vi "FGGA Serial Data Server & Recordingv5.0_10Hz_Scroll_Pump.vi"(0 "VISA resource name out":refnum<visa-resource-name>, 11 "error IO":errorcluster) -> ()   [LabVIEW 2014]
uses:
  <vilib>/Platform/TimedLoop/XDataNode/timing_clust.ctl
  <vilib>/Platform/TimedLoop/XDataNode/nitl_modes.ctl
  <vilib>/Platform/TimedLoop/XDataNode/wakeup.ctl
  C:/Program Files (x86)/National Instruments/LabVIEW 2014/examples/Data Communication/Network Streams/Simple Network Streams/support/Network Stream Command.ctl
  <vilib>/Utility/error.llb/whitespace.ctl
  <vilib>/Utility/tcp.llb/UDP Multicast Write-Only Open.vi
  <vilib>/Instr/_visa.llb/VISA Configure Serial Port (Instr).vi
  <vilib>/platform/TimedLoop/XDataNode/XDataNode.xnode
  <vilib>/Platform/TimedLoop/XDataNode/XDNodeRunTimeDep.lvlib
panel:
  out "FLOW ALL OFF":bool
  out "LOW FLOW MASTER SWITCH":bool
  out "HIGH FLOW MASTER SWITCH":bool
  out "UDP_ASCII_File":string
  out "V12":bool
  out "V11":bool
  out "V10":bool
  out "FGGA Pump":bool
  out "Flight Number":string
  out "Stop File Write":bool
  out "Default file name":string
  out "MFC":dbl[](array[numeric])
  out "FGGA restart":bool
  out "V4":bool
  out "V3":bool
  out "V2":bool
  out "V1":bool
  out "error out 2":errorcluster
  out "error out":errorcluster
  in  "MFC_1 SLPM set value":dbl
  out "Value Read":string
  out "status":bool
  in  "VISA resource name":refnum<visa-resource-name>="ASRL3::INSTR"
  in  "timeout (10sec) 2":u32=3000
  out "Labview_Viewer_UDP_Error_Out":errorcluster
  in  "Clear Display\nErrors":bool
  out "Data Processing":bool
  out "TCP Binary Packet":string
  out "UDP Time Stamp Offset":i32=1
  out "Data String":string
  out "UDP_ACSII_Out":string
  out "Serial error out":errorcluster
  out "SEPTIC TCP Error Out":errorcluster
  out "TCP packet\nSend To SEPTIC":bool
  out "FISH TCP Error Out":errorcluster
  out "TCP packet\nSend To FISH":bool
  out "UDP_Pack_num":u32
  out "UDP_Out Status":bool
  out "UDP_Out_Error Out":errorcluster
  out "Data Array":string[](array[string])
  out "RAW DATA":string
  in  "stop":bool
  out "Number of times \nRead time out":u32
  out "Loop count":i32
  # "Date"
  # "Time"
  # "CH4"
  # "CO2"
  # "H2O"
  # "Cell Pressure"
  # "Cell Temperature"
  # "Spectral Flag"
  # "Ring Down Time (Laser A)"
  # "Ring Down Time (Laser B)"
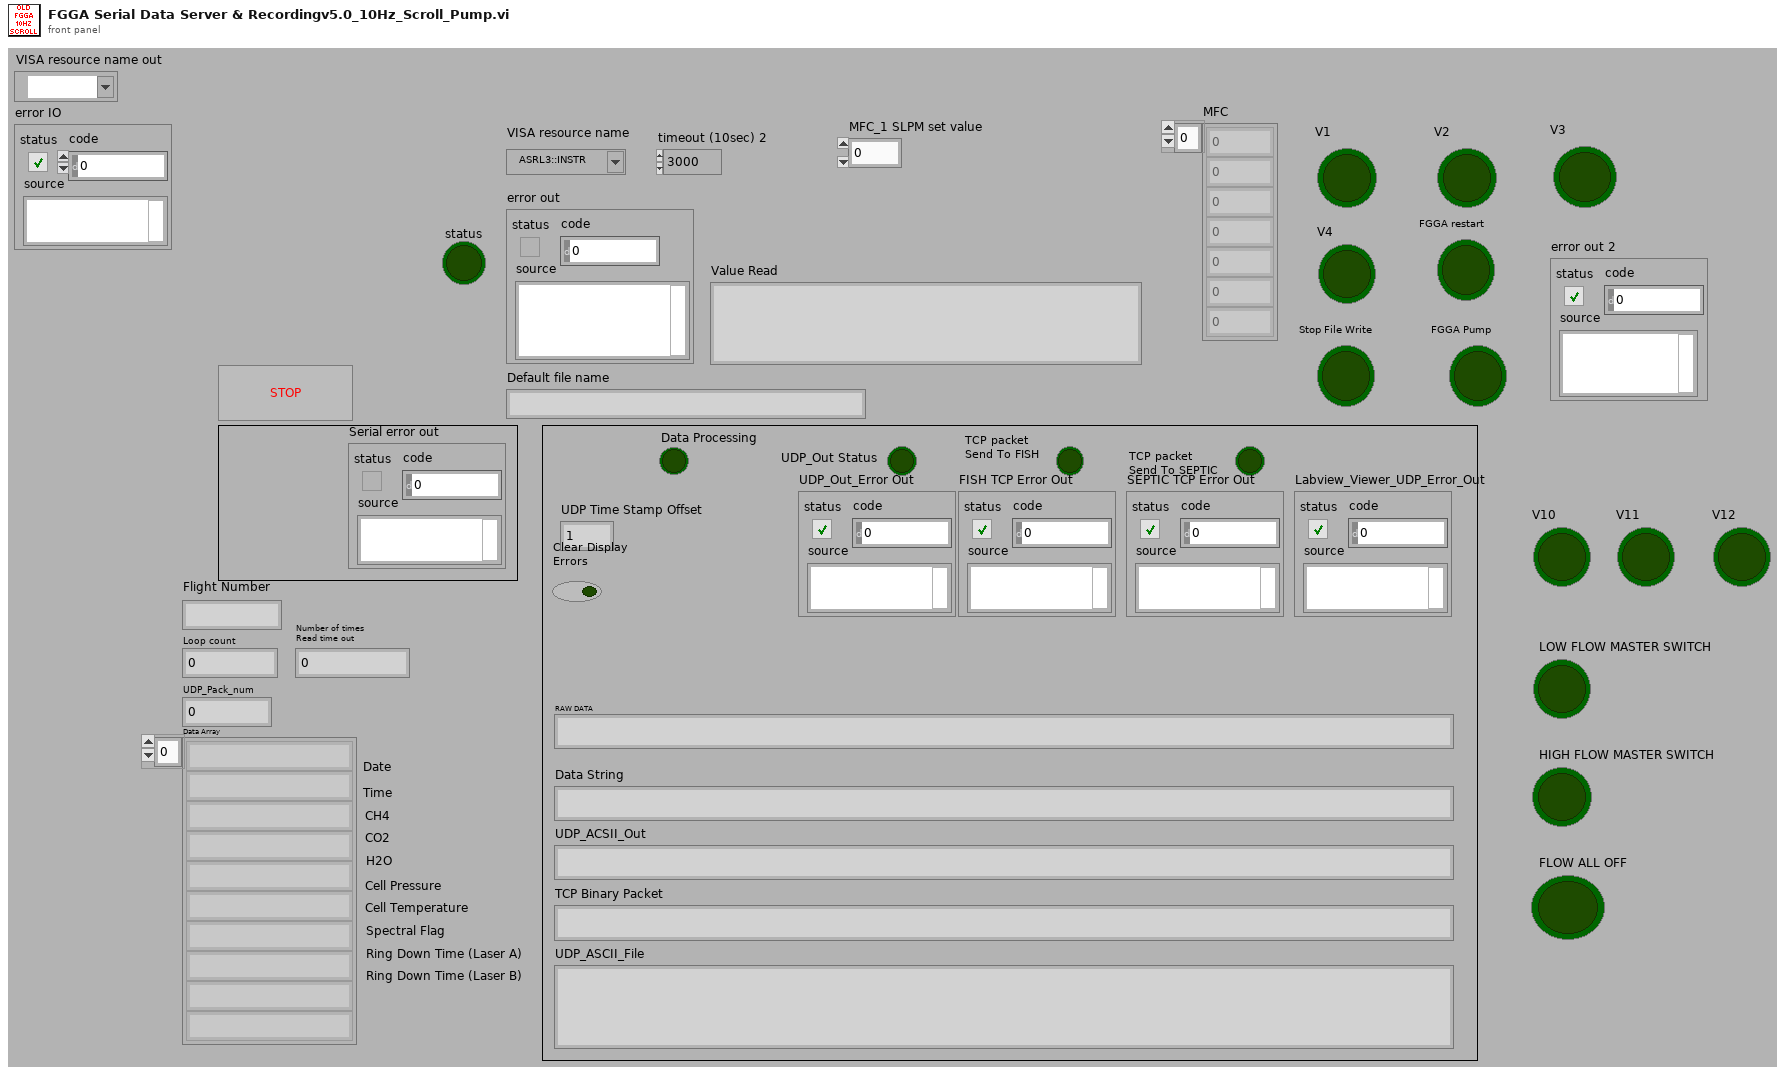
[diagram p1: front panel]
types:
  T1 = typedef "XDNodeRunTimeDep.lvlib/timing_clust.ctl" = cluster{"Expected End [f-1]":u64, "Actual End [f-1]":u64, "Finished Late? [f-1]":bool, "Expected End [i-1]":u64, "Actual End [i-1]":u64, "Finished Late? [i-1]":bool, "Expected Start [i]":u64, "Actual Start [i]":u64, "Expected Start [f]":u64, "Actual Start [f]":u64, "Source Name":string, "Structure Name":string, "Period":i64, "Deadline":i64, "Offset":i64, "Start":i64, "Priority":i32, "Timeout":i32, "Mode":T2, "Wakeup Reason":T3, "Error":errorcluster, "Source Type":string, "Secondary Source Type":string, "Global End Time":u64, "Global Start Time":u64, "Frame Duration":u64, "Iteration Duration":u64, "Assigned CPU":i32, "I/O Scan Engine Mode":u32}
  T2 = typedef "XDNodeRunTimeDep.lvlib/nitl_modes.ctl" = enum32{"No Change", "Process missed periods, maintain original phase", "Discard missed periods, maintain original phase", "Process missed periods, ignore original phase", "Discard missed periods, ignore original phase"}
  T3 = typedef "XDNodeRunTimeDep.lvlib/wakeup.ctl" = enum32{"Normal", "Aborted", "Asynchronous wakeup", "Timing source error", "Timed loop error", "Timeout"}
  T4 = typedef "Network Stream Command.ctl" = cluster{"Message":string, "Message Data":variant}
  T5 = enum16{"open", "replace", "create", "open or create", "replace or create", "replace or create with confirmation"}
  T6 = typedef "whitespace.ctl" = u16
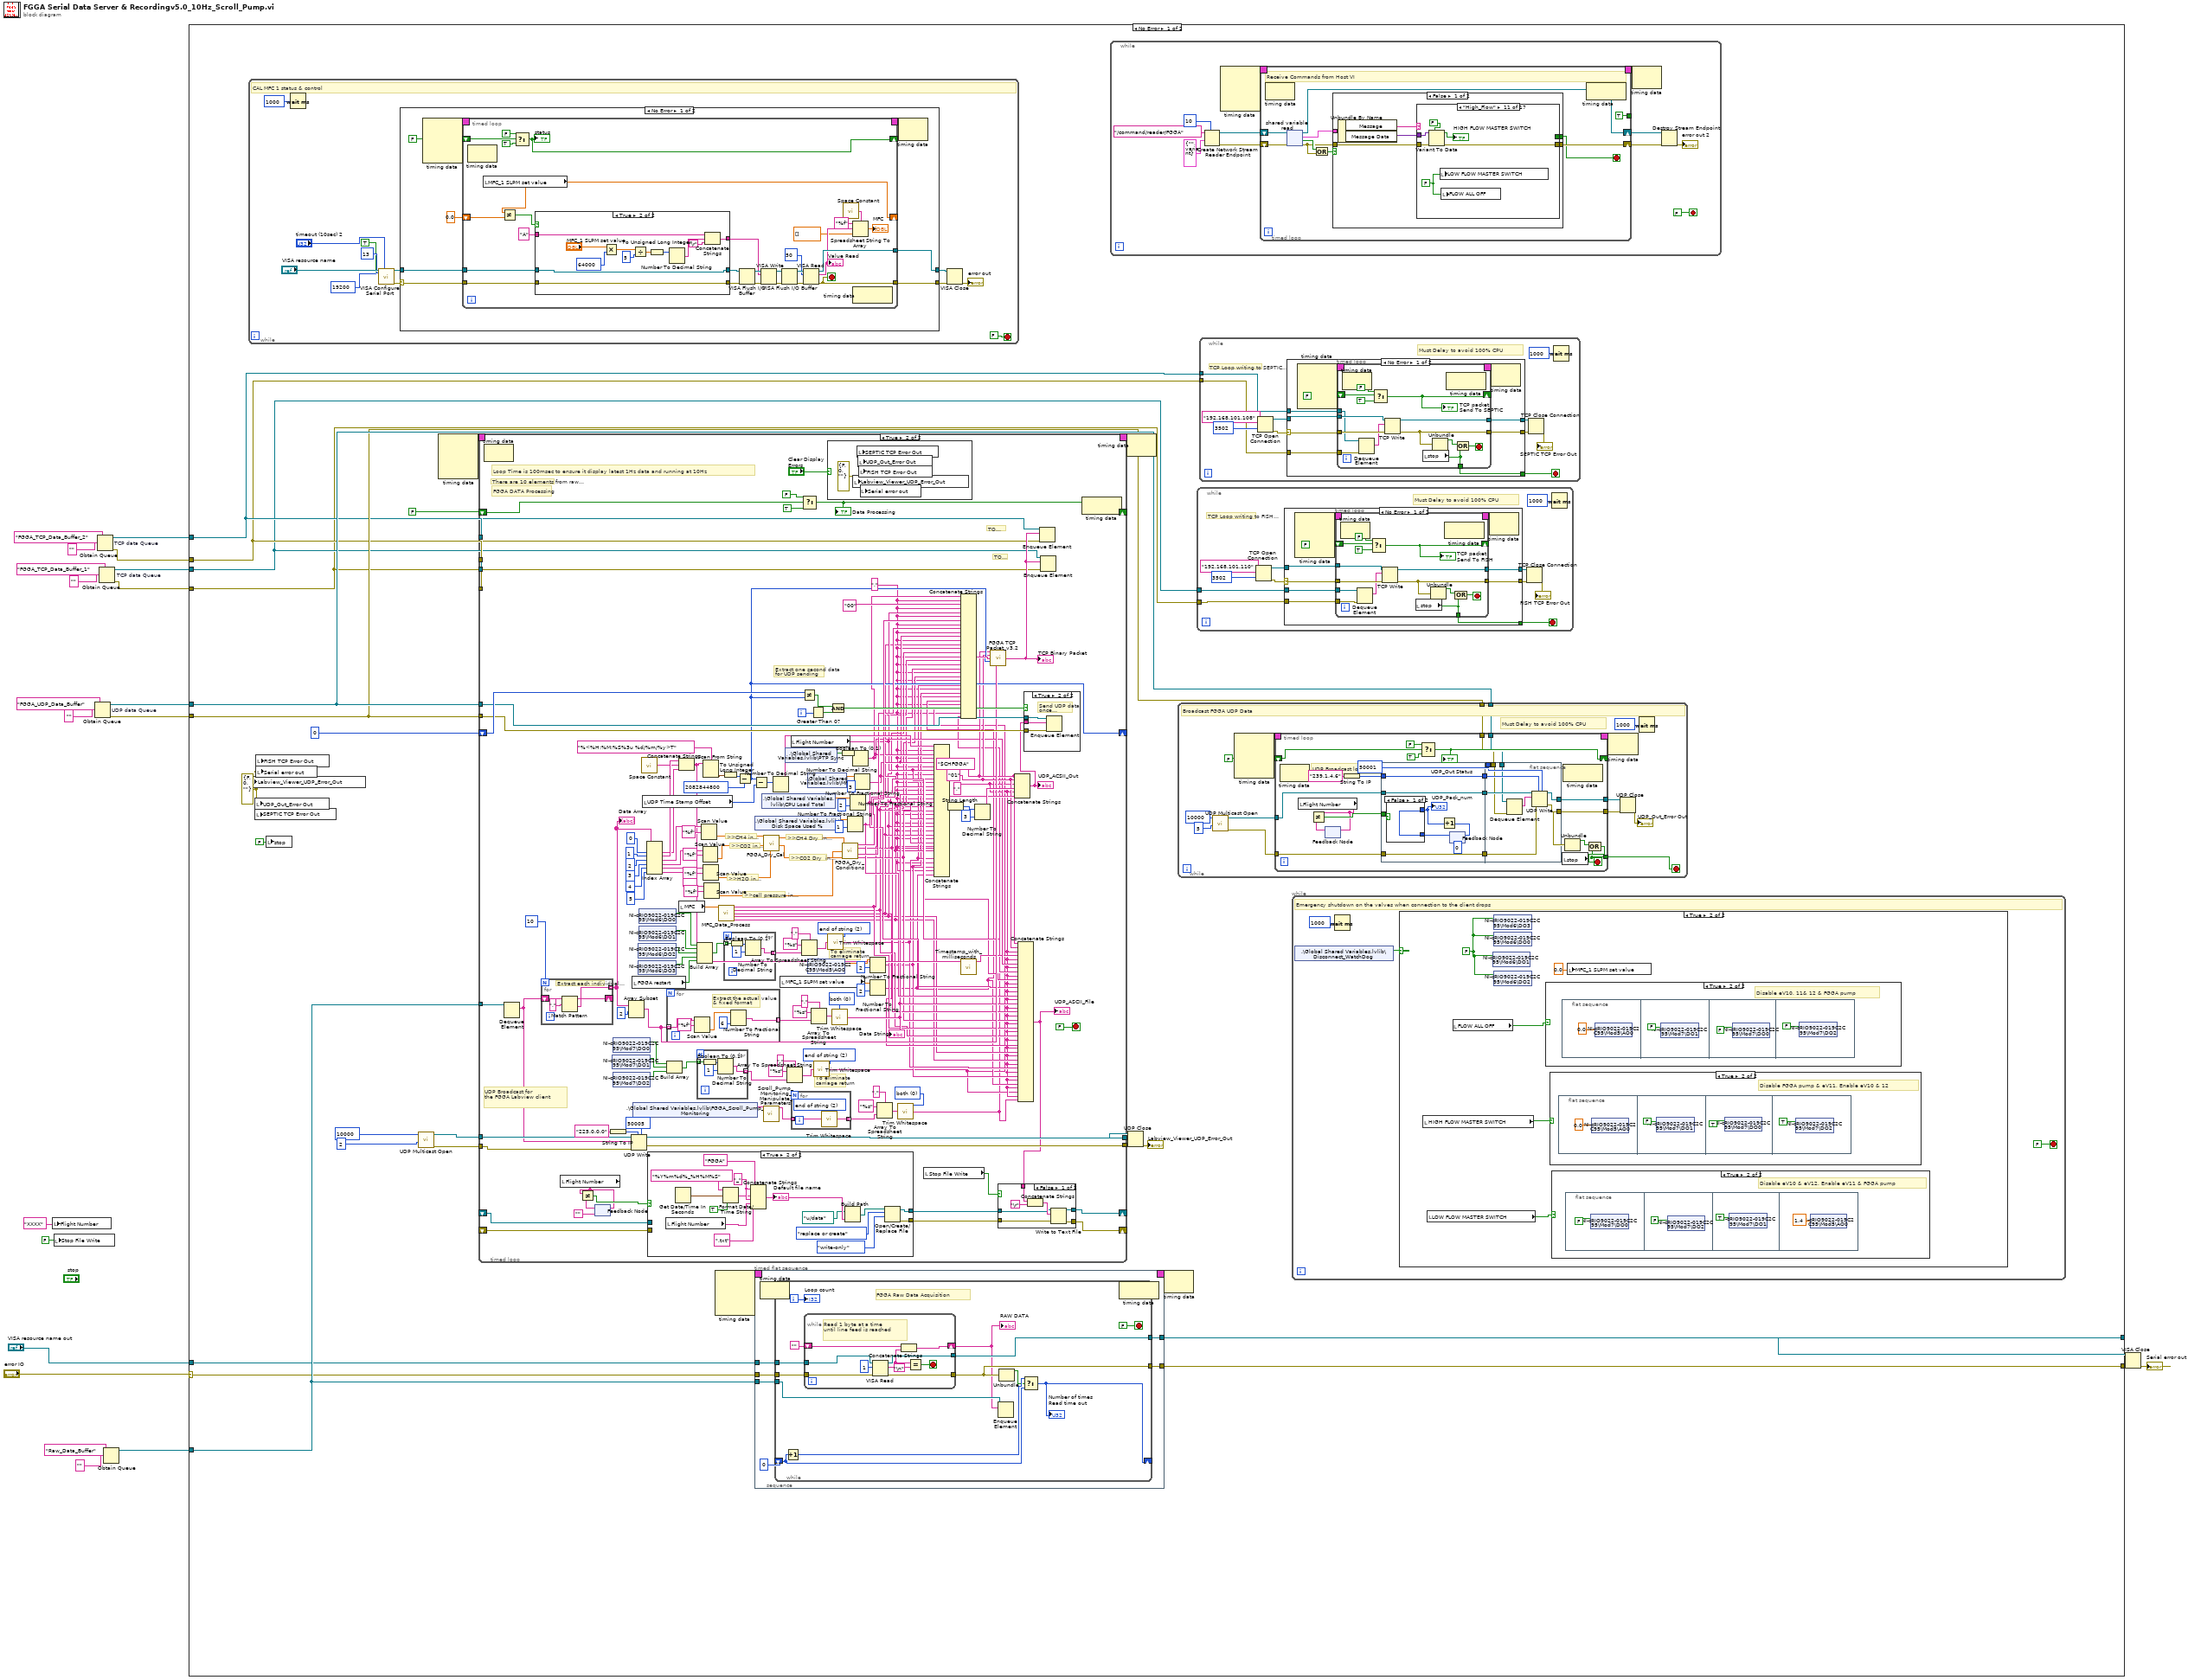
[diagram p0: block diagram]
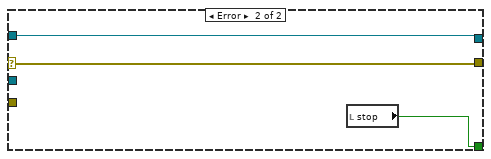
[diagram p6: hidden frame]
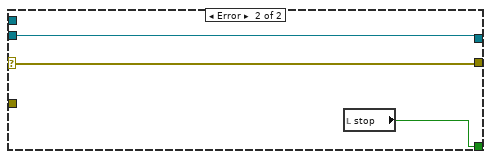
[diagram p7: hidden frame]
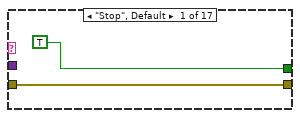
[diagram p8: hidden frame]
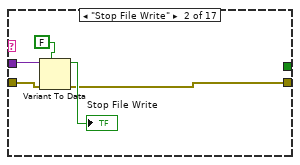
[diagram p9: hidden frame]
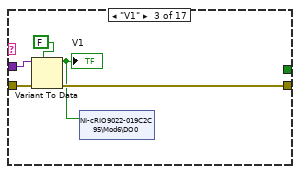
[diagram p10: hidden frame]
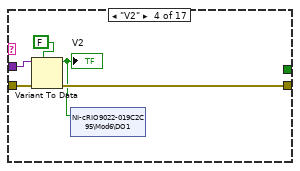
[diagram p11: hidden frame]
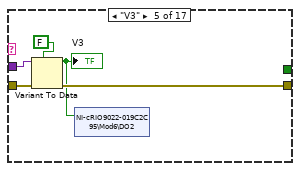
[diagram p12: hidden frame]
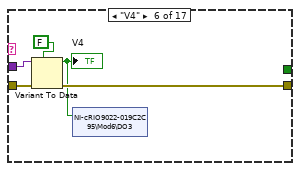
[diagram p13: hidden frame]
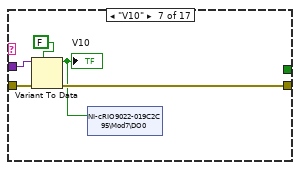
[diagram p14: hidden frame]
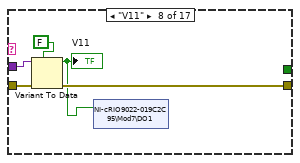
[diagram p15: hidden frame]
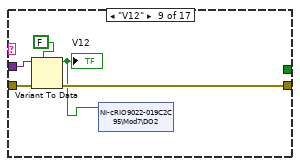
[diagram p16: hidden frame]
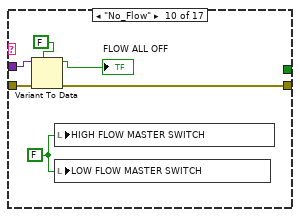
[diagram p17: hidden frame]
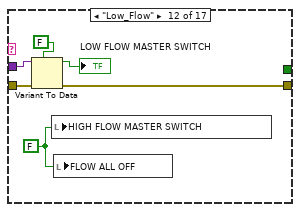
[diagram p18: hidden frame]
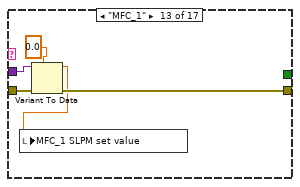
[diagram p19: hidden frame]
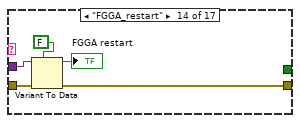
[diagram p20: hidden frame]
diagram:
  n1 = local write "Flight Number"("XXXX" ("Flight Number")) -> ()
  n2 = local write "Stop File Write"(FALSE ("Stop File Write")) -> ()
  n3 = Obtain Queue "UDP data Queue"(name (unnamed)="FGGA_UDP_Data_Buffer", element data type="") -> (queue out=w14:refnum<queue>, error out=w13:errorcluster)  [unwired: 3 in, 1 out]
  n4 = Obtain Queue "TCP data Queue"(name (unnamed)="FGGA_TCP_Data_Buffer_2", element data type="") -> (queue out=w8:refnum<queue>, error out=w7:errorcluster)  [unwired: 3 in, 1 out]
  n5 = Obtain Queue "TCP data Queue"(name (unnamed)="FGGA_TCP_Data_Buffer_1", element data type="") -> (queue out=w6:refnum<queue>, error out=w5:errorcluster)  [unwired: 3 in, 1 out]
  n6 = Obtain Queue(name (unnamed)="Raw_Data_Buffer", element data type="") -> (queue out=w20:refnum<queue>)  [unwired: 3 in, 2 out]
  n7 = case shown="No Error" "error IO" {
    selector: "error IO" -> [w25 w647]
    tunnel: "VISA resource name out" -> [w26 w648]
    tunnel: [w47 w648] -> w17
    tunnel: [w48 w647] -> w18
    tunnel: w20 -> [w44 _]
    tunnel: w14 -> [w42 _]
    tunnel: w13 -> [w41 _]
    tunnel: w8 -> [w40 _]
    tunnel: w7 -> [w39 _]
    tunnel: w6 -> [w38 _]
    tunnel: w5 -> [w37 _]
    frame No Error {
      w28 = errorcluster {"status"=FALSE, "code"=0, "source"=""} ("UDP Error Out")
      n8 = while {
        stop <- FALSE stop-if-true
        # "CAL MFC 1 status & control"
        n9 = Wait (ms)(milliseconds to wait=u32 1000) -> ()  [unwired: 1 out]
        n10 = call-poly "VISA Configure Serial Port"("VISA resource name"="VISA resource name", "timeout (10sec)"="timeout (10sec) 2", "termination char\n(0xA = '\\n' = LF)"=u8 13 ("termination char\n(0xA = '\\n' = LF)"), "Enable Termination\nChar (T)"=TRUE ("Enable Termination\nChar (T)"), "baud rate (9600)"=u32 19200) -> ("VISA resource name out"=w323:refnum<visa-resource-name>, "error out"=w319:errorcluster)  [unwired: 9 in]
        n11 = case shown="No Error" w319 {
          selector: w319 -> [w330 w380]
          tunnel: w323 -> [w331 w381]
          tunnel: [w329 w381] -> w322
          tunnel: [w328 w380] -> w321
          frame No Error {
            n12 = node-c288() -> (w326:T1)  [unwired: 4 in]
            n13 = timed-loop {
              tunnel: w331 -> [w354]
              tunnel: w330 -> [w352]
              tunnel: [w345] -> w329
              tunnel: [w340] -> w328
              shift-right: [w341] -> _
              shift-left: FALSE -> [w344]
              timing: w326 -> [_]
              timing-out: [_] -> w325
              shift-right: [w332] -> _
              shift-left: 0.0 -> [w334]
              stop <- w340 stop-if-true
              n14 = node-c288() -> ()  [unwired: 1 in, 1 out]
              n15 = local read "MFC_1 SLPM set value"() -> (w332:dbl)
              n16 = Not Equal?(x=w332, y=w334) -> (x != y?=w333:bool)
              n17 = Select(t=FALSE, s=w344, f=TRUE) -> (s? t:f=w341:bool)
              "status" <- w341
              n18 = case shown="True" w333 {
                tunnel: w354 -> [w362 w377]
                tunnel: [w362 w377] -> w353
                tunnel: w352 -> [w361 w376]
                tunnel: [w361 w376] -> w351
                tunnel: "A" -> [w365 w369]
                tunnel: [w363 w366] -> w349
                frame False {
                  n19 = Concatenate Strings(w365, "\r") -> (w363:string)
                }
                frame True {
                  n20 = Multiply(x="MFC_1 SLPM set value", y=u32 64000) -> (x*y=w373:dbl)
                  n21 = Divide(x=w373, y=u32 5) -> (x/y=w371:dbl)
                  n22 = To Unsigned Long Integer(number=w371) -> (unsigned 32bit integer=w370:u32)
                  n23 = Number To Decimal String(number=w370) -> (decimal integer string=w368:string)  [unwired: 1 in]
                  n24 = Concatenate Strings(w369, w368, "\r") -> (w366:string)
                }
              }
              n25 = VISA Flush I/O Buffer(VISA resource name=w353, error in (no error)=w351) -> (VISA resource name out=w356:refnum<visa-resource-name>, error out=w355:errorcluster)  [unwired: 1 in]
              n26 = VISA Write(VISA resource name=w356, write buffer=w349, error in (no error)=w355) -> (VISA resource name out=w348:refnum<visa-resource-name>, error out=w347:errorcluster)  [unwired: 1 out]
              n27 = VISA Flush I/O Buffer(VISA resource name=w348, error in (no error)=w347) -> (VISA resource name out=w358:refnum<visa-resource-name>, error out=w357:errorcluster)  [unwired: 1 in]
              n28 = VISA Read(VISA resource name=w358, byte count=u32 50, error in (no error)=w357) -> (VISA resource name out=w345:refnum<visa-resource-name>, read buffer=w339:string, error out=w340:errorcluster)  [unwired: 1 out]
              "Value Read" <- w339
              n29 = call <vilib>:"Space Constant.vi"() -> ("String"=w338:string)
              n30 = Spreadsheet String To Array(delimiter (Tab)=w338, format string="%f", spreadsheet string=w339, array type (2D Dbl)=dbl[] []) -> (array=→"MFC":dbl[])
              n31 = node-c288() -> ()  [unwired: 1 in, 1 out]
            }
            n32 = node-c288(w325) -> ()  [unwired: 1 out]
          }
          frame Error {
          }
        }
        n33 = VISA Close(VISA resource name=w322, error in (no error)=w321) -> (error out=→"error out":errorcluster)
      }
      n34 = local write "Labview_Viewer_UDP_Error_Out"(w28) -> ()
      n35 = local write "UDP_Out_Error Out"(w28) -> ()
      n36 = local write "SEPTIC TCP Error Out"(w28) -> ()
      n37 = local write "FISH TCP Error Out"(w28) -> ()
      n38 = local write "Serial error out"(w28) -> ()
      n39 = local write "stop"(FALSE ("stop")) -> ()
      n40 = call-poly <vilib>:"UDP Multicast Open.vi"("time-to-live (1)"=u16 2, "port"=u16 10000) -> ("error out"=w32:errorcluster, "connection ID"=w33:refnum<k16>)  [unwired: 8 in]
      n41 = node-c288() -> (w46:T1)  [unwired: 4 in]
      n42 = timed-loop {
        timing: w46 -> [_]
        timing-out: [_] -> w45
        tunnel: w44 -> [w592]
        tunnel: w42 -> [w551]
        tunnel: w41 -> [w550]
        shift-right: [w483] -> _
        shift-left: u32 0 -> [w554]
        tunnel: w40 -> [w547]
        tunnel: w39 -> [w546]
        tunnel: w38 -> [w545]
        tunnel: w37 -> [w544]
        shift-right: [w540] -> _
        shift-left: FALSE -> [w543]
        tunnel: w33 -> [w536]
        tunnel: w32 -> [w535]
        tunnel: [w534] -> w31
        tunnel: [w533] -> w30
        shift-right: [w522] -> _
        shift-left: _ -> [w515]
        shift-right: [w513] -> _
        shift-left: _ -> [w514]
        i -> [w553]
        stop <- FALSE stop-if-true
        w470 = T6 0 items=["both", "start of string", "end of string"] ("location (both)")
        w475 = T6 2 items=["both", "start of string", "end of string"] ("location (both)")
        w489 = T6 2 items=["both", "start of string", "end of string"] ("location (both)")
        w442 = ","
        w579 = T6 0 items=["both", "start of string", "end of string"] ("location (both)")
        w446 = ","
        w466 = "01"
        w467 = "$CHFGGA"
        # "To eliminate\ncarriage return"
        # "To eliminate\ncarriage return"
        # ">>cell pressure in torr>>"
        # "UDP Broadcast for\nthe FGGA Labview client"
        # "There are 10 elements from raw packet"
        # "TO SEPTIC"
        # "TO FISH"
        # "Extract one second data\nfor UDP sending"
        # ">>CO2 Dry  in ppm>>"
        # ">>CH4 Dry  in ppb>>"
        # ">>H2O in ppm>>"
        # ">>CO2 in ppm>>"
        # ">>CH4 in ppm>>"
        # "Loop Time is 100msec to ensure it display latest 1Hz data and running at 10Hz"
        # "FGGA DATA Processing"
        n43 = node-c288() -> ()  [unwired: 1 in, 1 out]
        n44 = Dequeue Element(queue=w592) -> (element=w532:string)  [unwired: 2 in, 3 out]
        n45 = for {
          N: 10 -> [_]
          shift-right: [w641] -> _
          shift-left: w532 -> [w639]
          tunnel: [w640] -> w584 mode=indexing
          # "Extract each individual param"
          n46 = Match Pattern(string=w639, regular expression=",") -> (before substring=w640:string, after substring=w641:string)  [unwired: 1 in, 2 out]
        }
        "Data Array" <- w584
        n47 = local read "Flight Number"() -> (w512:string)
        n48 = feedback #1("" ("Flight Number")) -> (w520:string)
        n49 = Not Equal?(x=w512, y=w520) -> (x != y?=w518:bool)
        n50 = feedback-in #1(w512) -> ()
        n51 = String To IP(1:"225.0.0.0" ("name")) -> (0:w537:u32)
        n52 = shared-variable "NI-cRIO9022-019C2C95\\Mod7\\DO1"() -> (w480:bool)  [unwired: 1 in, 1 out]
        n53 = shared-variable "NI-cRIO9022-019C2C95\\Mod7\\DO0"() -> (w481:bool)  [unwired: 1 in, 1 out]
        n54 = shared-variable "NI-cRIO9022-019C2C95\\Mod7\\DO2"() -> (w479:bool)  [unwired: 1 in, 1 out]
        n55 = Array Subset(array=w584, index=2) -> (w549:string[])  [unwired: 1 in]
        n56 = UDP Write(address=w537, port or service name=u16 50005, connection ID=w536, data in=w532, 8:w535) -> (error out=w533:errorcluster, 3:w534:refnum<k16>)  [unwired: 1 in]
        n57 = local read "FGGA restart"() -> (w497:bool)
        n58 = shared-variable ".\\Global Shared Variables.lvlib\\FGGA_Scroll_Pump_Monitoring"() -> (w445:string[])  [unwired: 1 in, 1 out]
        n59 = shared-variable "NI-cRIO9022-019C2C95\\Mod6\\DO2"() -> (w503:bool)  [unwired: 1 in, 1 out]
        n60 = shared-variable "NI-cRIO9022-019C2C95\\Mod6\\DO3"() -> (w502:bool)  [unwired: 1 in, 1 out]
        n61 = shared-variable "NI-cRIO9022-019C2C95\\Mod6\\DO0"() -> (w505:bool)  [unwired: 1 in, 1 out]
        n62 = shared-variable "NI-cRIO9022-019C2C95\\Mod6\\DO1"() -> (w504:bool)  [unwired: 1 in, 1 out]
        n63 = call <vilib>:"Space Constant.vi"() -> ("String"=w563:string)
        n64 = local read "UDP Time Stamp Offset"() -> (w488:i32)
        n65 = Index Array(array=w584, index #1=0 ("index"), index #2=1 ("index"), index #3=2 ("index"), index #4=3 ("index"), index #5=4 ("index"), index #6=5 ("index")) -> (element #1=w562:string, element #2=w564:string, element #3=w568:string, element #4=w567:string, element #5=w566:string, element #6=w527:string)
        n66 = case shown="True" w518 {
          tunnel: [w605 w607] -> w517
          tunnel: [w604 w606] -> w516
          tunnel: w515 -> [w605 _]
          tunnel: w514 -> [w604 _]
          frame False {
          }
          frame True {
            w613 = "_" ("string")
            n67 = local read "Flight Number"() -> (w620:string)
            n68 = Get Date/Time In Seconds() -> (seconds since 1Jan1904=w608:timestamp)
            n69 = Format Date/Time String(time format string (%c)="%Y%m%d%_%H%M%S", seconds (now)=w608, UTC format=TRUE) -> (date/time string=w610:string)
            n70 = Concatenate Strings("FGGA" ("string"), w613, w610, w613, w620, ".txt" ("string")) -> (w615:string)
            "Default file name" <- w615
            n71 = Build Path(base path=path "u:/data", name or relative path=w615) -> (appended path=w619:path)
            n72 = Open/Create/Replace File(file path (use dialog)=w619, operation (0:open)=T5."replace or create", access (0:read/write)=enum16{"read/write", "read-only", "write-only"}."write-only") -> (refnum out=w607:refnum<file>, error out=w606:errorcluster)  [unwired: 3 in, 1 out]
          }
        }
        n73 = for {
          tunnel: w549 -> [w637] mode=indexing
          tunnel: [w634] -> w577 mode=indexing
          # "Extract the actual value\n& fixed format"
          n74 = Scan Value(string=w637, format string="%f") -> (value=w635:dbl)  [unwired: 1 in, 1 out]
          n75 = Number To Fractional String(number=w635, precision (6)=i16 6) -> (F-format string=w634:string)  [unwired: 2 in]
        }
        n76 = Build Array(w481, w480, w479) -> (w482:bool[])
        n77 = Concatenate Strings(w564, w563, w562) -> (w462:string)
        n78 = local read "MFC"() -> (w523:dbl[])
        n79 = for {
          tunnel: w482 -> [w598] mode=indexing
          tunnel: [w597] -> w474 mode=indexing
          n80 = Boolean To (0,1)(Boolean=w598) -> (0, 1=w599:i16)
          n81 = Number To Decimal String(number=w599, width (-)=i16 1) -> (decimal integer string=w597:string)
        }
        n82 = Build Array(w505, w504, w503, w502, w497) -> (w501:bool[])
        n83 = Scan Value(string=w568, format string="%f") -> (value=w570:dbl)  [unwired: 1 in, 1 out]
        n84 = Scan Value(string=w567, format string="%f") -> (value=w569:dbl)  [unwired: 1 in, 1 out]
        n85 = Scan From String(format string="%<%H:%M:%S%3u %d/%m/%y>T", input string=w462) -> (output 1=w559:timestamp)  [unwired: 3 in, 3 out]
        n86 = Scan Value(string=w566, format string="%f") -> (value=w524:dbl)  [unwired: 1 in, 1 out]
        n87 = Scan Value(string=w527, format string="%f") -> (value=w525:dbl)  [unwired: 1 in, 1 out]
        n88 = call "MFC_Data_Process.vi"("MFC"=w523) -> ("MFC Absolute Pressure"=w454:string, "MFC Temperature"=w453:string, "MFC Volumetric Flow"=w452:string, "MFC Mass Flow"=w451:string, "MFC Set Point"=w450:string)  [unwired: 10 in]
        n89 = To Unsigned Long Integer(number=w559) -> (unsigned 32bit integer=w560:u32)
        n90 = for {
          tunnel: w501 -> [w602] mode=indexing
          tunnel: [w601] -> w498 mode=indexing
          n91 = Boolean To (0,1)(Boolean=w602) -> (0, 1=w603:i16)
          n92 = Number To Decimal String(number=w603, width (-)=i16 1) -> (decimal integer string=w601:string)
        }
        n93 = Subtract(x=w560, y=u32 2082844800) -> (x-y=w483:u32)
        n94 = Subtract(x=w483, y=w488) -> (x-y=w557:u32)
        n95 = shared-variable ".\\Global Shared Variables.lvlib\\Disk Space Used %"() -> (w491:dbl)  [unwired: 1 in, 1 out]
        n96 = shared-variable ".\\Global Shared Variables.lvlib\\CPU Load Total"() -> (w511:dbl)  [unwired: 1 in, 1 out]
        n97 = call "Scroll_Pump_Monitoring_Manipulate_Parameters.vi"("FGGA_Scroll_Pump\nMonitoring_Input"=w445) -> ("output array"=w444:string[])  [unwired: 14 in]
        n98 = call "FGGA_Dry_Cal.vi"("H2O"=w524, "CO2_Wet"=w569, "CH4_Wet"=w570) -> ("CO2_Dry"=w529:dbl, "CH4_Dry"=w531:dbl)  [unwired: 7 in]
        n99 = Number To Decimal String(number=w557) -> (decimal integer string=w558:string)  [unwired: 1 in]
        n100 = local read "MFC_1 SLPM set value"() -> (w493:dbl)
        n101 = shared-variable ".\\Global Shared Variables.lvlib\\PTP Sync"() -> (w506:bool)  [unwired: 1 in, 1 out]
        n102 = Array To Spreadsheet String(delimiter (Tab)=",", array=w474, 3:"%s" ("format string")) -> (spreadsheet string=w476:string)
        n103 = local read "Flight Number"() -> (w460:string)
        n104 = for {
          tunnel: w444 -> [w595] mode=indexing
          tunnel: [w594] -> w469 mode=indexing
          w593 = T6 2 items=["both", "start of string", "end of string"] ("location (both)")
          n105 = call <vilib>:"Trim Whitespace.vi"("string"=w595, "location (both)"=w593) -> ("trimmed string"=w594:string)
        }
        n106 = Array To Spreadsheet String(delimiter (Tab)=",", array=w498, 3:"%s" ("format string")) -> (spreadsheet string=w490:string)
        n107 = Select(t=FALSE, s=w543, f=TRUE) -> (s? t:f=w540:bool)
        "Data Processing" <- w540
        n108 = Not Equal?(x=w554, y=w483) -> (x != y?=w555:bool)
        n109 = shared-variable ".\\Global Shared Variables.lvlib\\MFM"() -> (w509:dbl)  [unwired: 1 in, 1 out]
        n110 = shared-variable "NI-cRIO9022-019C2C95\\Mod5\\AO0"() -> (w495:dbl)  [unwired: 1 in, 1 out]
        n111 = Greater Than 0?(x=w553) -> (x > 0?=w556:bool)
        n112 = Array To Spreadsheet String(delimiter (Tab)=",", array=w577, 3:"%s" ("format string")) -> (spreadsheet string=w578:string)
        n113 = call <vilib>:"Trim Whitespace.vi"("string"=w476, "location (both)"=w475) -> ("trimmed string"=w443:string)
        n114 = case shown="True" "Clear Display\nErrors" {
          frame False {
          }
          frame True {
            w630 = errorcluster {"status"=FALSE, "code"=0, "source"=""} ("UDP Error Out")
            n115 = local write "Labview_Viewer_UDP_Error_Out"(w630) -> ()
            n116 = local write "SEPTIC TCP Error Out"(w630) -> ()
            n117 = local write "UDP_Out_Error Out"(w630) -> ()
            n118 = local write "FISH TCP Error Out"(w630) -> ()
            n119 = local write "Serial error out"(w630) -> ()
          }
        }
        n120 = call <vilib>:"Trim Whitespace.vi"("string"=w490, "location (both)"=w489) -> ("trimmed string"=w449:string)
        n121 = call <vilib>:"Trim Whitespace.vi"("string"=w578, "location (both)"=w579) -> ("trimmed string"=w457:string)
        "Data String" <- w457
        n122 = Compound Arithmetic op=AND(w555, w556) -> (w552:bool)
        n123 = Boolean To (0,1)(Boolean=w506) -> (0, 1=w507:i16)
        n124 = call "FGGA_Dry_Conditions.vi"("CH4_Dry"=w531, "Pressure"=w525, "CO2_Dry"=w529) -> ("CH4_Dry_TCP"=w487:string, "CH4_Dry_UDP"=w456:string, "CO2_Dry_TCP"=w486:string, "CO2_Dry_UDP"=w455:string)  [unwired: 9 in]
        n125 = Number To Fractional String(number=w491, precision (6)=i16 1) -> (F-format string=w458:string)  [unwired: 2 in]
        n126 = Number To Fractional String(number=w511, precision (6)=i16 2) -> (F-format string=w459:string)  [unwired: 2 in]
        n127 = Number To Decimal String(number=w507) -> (decimal integer string=w464:string)  [unwired: 1 in]
        n128 = Number To Fractional String(number=w509, precision (6)=i16 3) -> (F-format string=w461:string)  [unwired: 2 in]
        n129 = Number To Fractional String(number=w495, precision (6)=i16 2) -> (F-format string=w448:string)  [unwired: 2 in]
        n130 = Number To Fractional String(number=w493, precision (6)=i16 2) -> (F-format string=w447:string)  [unwired: 2 in]
        n131 = Array To Spreadsheet String(delimiter (Tab)=",", array=w469, 3:"%s" ("format string")) -> (spreadsheet string=w471:string)
        n132 = call <vilib>:"Trim Whitespace.vi"("string"=w471, "location (both)"=w470) -> ("trimmed string"=w441:string)
        n133 = local read "Stop File Write"() -> (w521:bool)
        n134 = Concatenate Strings(w558, w442, w464, w442, w461, w442, w460, w442, w459, w442, w458, w442, w457, w442, w456, w442, w455, w442, w454, w442, w453, w442, w452, w442, w451, w442, w450, w442, w449, w442, w448, w442, w447) -> (w586:string)
        n135 = String Length(string=w586) -> (length=w589:i32)
        n136 = Concatenate Strings(w464, w442, "00", w442, w460, w442, w487, w442, w486, w442, w461, w442, w454, w442, w453, w442, w452, w442, w451, w442, w450, w442, w449, w442, w448, w442, w447, w442, w443, w442, w441) -> (w485:string)
        n137 = call "Timestamp_with_milliseconds.vi"("Input Time"=w462) -> ("Output Time"=w463:string)  [unwired: 14 in]
        n138 = Number To Decimal String(number=w589, width (-)=i16 3) -> (decimal integer string=w587:string)
        n139 = call "FGGA TCP Packet_v3.2.vi"("ID"=w467, "Version"=w466, "TCP Packet In"=w485, "utc_time"=w483, "Data Array"=w549) -> ("TCP Binary Packet"=w548:string)  [unwired: 10 in]
        "TCP Binary Packet" <- w548
        n140 = Concatenate Strings(w467, w466, w446, w587, w446, w586) -> (w468:string)
        "UDP_ACSII_Out" <- w468
        n141 = Concatenate Strings(w467, w466, w446, w463, w446, w464, w446, w461, w446, w460, w446, w459, w446, w458, w446, w457, w446, w456, w446, w455, w446, w454, w446, w453, w446, w452, w446, w451, w446, w450, w446, w449, w446, w448, w446, w447, w446, w443, w446, w441) -> (w465:string)
        "UDP_ASCII_File" <- w465
        n142 = case shown="False" w521 {
          tunnel: w465 -> [w627 _]
          tunnel: [w624 _] -> w522
          tunnel: w517 -> [w623 w629]
          tunnel: w516 -> [w622 w628]
          tunnel: [w621 _] -> w513
          frame False {
            n143 = Concatenate Strings(w627, "\r") -> (w625:string)
            n144 = Write to Text File(file (use dialog)=w623, text=w625, error in=w622) -> (refnum out=w624:refnum<file>, error out=w621:errorcluster)  [unwired: 2 out]
          }
          frame True {
            n145 = Close File(refnum=w629, error in=w628) -> ()  [unwired: 2 out]
          }
        }
        n146 = case shown="True" w552 {
          tunnel: w468 -> [_ w633]
          tunnel: w551 -> [_ w632]
          tunnel: w550 -> [_ w631]
          frame False {
          }
          frame True {
            # "Send UDP data once\na second"
            n147 = Enqueue Element(queue=w632, element=w633, error in (no error)=w631) -> ()  [unwired: 1 in, 3 out]
          }
        }
        n148 = Enqueue Element(queue=w547, element=w548, error in (no error)=w546) -> ()  [unwired: 1 in, 3 out]
        n149 = Enqueue Element(queue=w545, element=w548, error in (no error)=w544) -> ()  [unwired: 1 in, 3 out]
        n150 = node-c288() -> ()  [unwired: 1 in, 1 out]
      }
      n151 = node-c288() -> (w24:T1)  [unwired: 4 in]
      n152 = timed-sequence {
        timing: w24 -> [_]
        timing-out: [_] -> w23
        tunnel: [w157] -> w48
        tunnel: [w156] -> w47
        tunnel: w44 -> [w155]
        tunnel: w26 -> [w154]
        tunnel: w25 -> [w153]
        n153 = timed-flat-sequence {
          tunnel: [w163] -> w157
          tunnel: [w162] -> w156
          tunnel: w155 -> [w160]
          tunnel: w154 -> [w159]
          tunnel: w153 -> [w158]
          n154 = node-c288() -> ()  [unwired: 1 in, 1 out]
          n155 = while {
            tunnel: w159 -> [w176]
            tunnel: w158 -> [w175]
            tunnel: [w174] -> w163
            shift-right: [w170] -> _
            shift-left: u32 0 -> [w171]
            tunnel: [w173] -> w162
            tunnel: w160 -> [w167]
            i -> [w172]
            stop <- FALSE stop-if-true
            # "FGGA Raw Data Acquisition"
            n156 = Increment(x=w171) -> (x+1=w169:u32)
            n157 = while {
              tunnel: [w186] -> w173
              tunnel: [w185] -> w174
              tunnel: w176 -> [w184]
              tunnel: w175 -> [w183]
              shift-right: [w181] -> w166
              shift-left: "" -> [w182]
              stop <- w178 stop-if-true
              # "Read 1 byte at a time \nuntil line feed is reached"
              n158 = VISA Read(VISA resource name=w184, byte count=u32 1, error in (no error)=w183) -> (VISA resource name out=w186:refnum<visa-resource-name>, read buffer=w180:string, error out=w185:errorcluster)  [unwired: 1 out]
              n159 = Concatenate Strings(w182, w180) -> (w181:string)
              n160 = Equal?(x=w180, y="\n") -> (x = y?=w178:bool)
            }
            "RAW DATA" <- w166
            n161 = Enqueue Element(queue=w167, element=w166) -> ()  [unwired: 2 in, 3 out]
            n162 = Unbundle(w174) -> ("status"=w165:bool)  [unwired: 2 out]
            n163 = Select(t=w169, s=w165, f=w171) -> (s? t:f=w170:u32)
            "Number of times \nRead time out" <- w170
            "Loop count" <- w172
          }
          n164 = node-c288() -> ()  [unwired: 1 in, 1 out]
        }
      }
      n165 = while {
        stop <- FALSE stop-if-true
        n166 = Create Network Stream Reader Endpoint(7:10 ("reader buffer size"), 9:T4 {"Message"="", "Message Data"=variant} ("Message Cluster"), 11:"/command/reader/FGGA" ("reader url")) -> (0:w197:errorcluster, 3:w198:refnum<k21>)  [unwired: 4 in]
        n167 = node-c288() -> (w192:T1)  [unwired: 4 in]
        n168 = timed-loop "Host->Target Command Reader" {
          shift-right: [w208] -> w195
          shift-left: w197 -> [w211]
          shift-right: [w209] -> w194
          shift-left: w198 -> [w210]
          tunnel: [TRUE] -> _
          timing: w192 -> [_]
          timing-out: [_] -> w191
          stop <- w202 stop-if-true
          # "Receive Commands from Host VI"
          n169 = node-c288() -> ()  [unwired: 1 in, 1 out]
          n170 = shared-variable-read(w210, w211) -> (w209:refnum<k21>, w204:errorcluster, w206:bool, w207:T4)  [unwired: 1 in]
          n171 = Or(x=w206, y=w204) -> (x .or. y?=w205:bool)
          n172 = case shown="False" w205 {
            selector: w205 -> [_ w308]
            tunnel: w204 -> [w219 w309]
            tunnel: [w218 w309] -> w208
            tunnel: w207 -> [w216 _]
            tunnel: [w217 w308] -> w202
            frame False {
              n173 = Unbundle By Name(w216) -> ("Message"=w215:string, "Message Data"=w214:variant)
              n174 = case shown="\"High_Flow\"" w215 {
                tunnel: w219 -> [w221 w226 w231 w236 w241 w246 w251 w256 w261 w267 w273 w279 w284 w289 w294 w302 w307]
                tunnel: [w221 w222 w230 w235 w240 w245 w250 w255 w260 w266 w272 w278 w283 w288 w293 w301 w306] -> w218
                tunnel: w214 -> [_ w225 w229 w234 w239 w244 w249 w254 w259 w265 w271 w277 w282 w287 w292 w300 w305]
                tunnel: [TRUE _ _ _ _ _ _ _ _ _ _ _ _ _ _ _ _] -> w217
                frame "Stop", Default {
                }
                frame "Stop File Write" {
                  n175 = Variant To Data(error in=w226, type=FALSE, Variant=w225) -> (data=→"Stop File Write":bool, error out=w222:errorcluster)
                }
                frame "V1" {
                  n176 = Variant To Data(error in=w231, type=FALSE, Variant=w229) -> (data=w227:bool, error out=w230:errorcluster)
                  "V1" <- w227
                  n177 = shared-variable "NI-cRIO9022-019C2C95\\Mod6\\DO0"(w227) -> ()  [unwired: 1 in, 1 out]
                }
                frame "V2" {
                  n178 = Variant To Data(error in=w236, type=FALSE, Variant=w234) -> (data=w232:bool, error out=w235:errorcluster)
                  "V2" <- w232
                  n179 = shared-variable "NI-cRIO9022-019C2C95\\Mod6\\DO1"(w232) -> ()  [unwired: 1 in, 1 out]
                }
                frame "V3" {
                  n180 = Variant To Data(error in=w241, type=FALSE, Variant=w239) -> (data=w237:bool, error out=w240:errorcluster)
                  "V3" <- w237
                  n181 = shared-variable "NI-cRIO9022-019C2C95\\Mod6\\DO2"(w237) -> ()  [unwired: 1 in, 1 out]
                }
                frame "V4" {
                  n182 = Variant To Data(error in=w246, type=FALSE, Variant=w244) -> (data=w242:bool, error out=w245:errorcluster)
                  "V4" <- w242
                  n183 = shared-variable "NI-cRIO9022-019C2C95\\Mod6\\DO3"(w242) -> ()  [unwired: 1 in, 1 out]
                }
                frame "V10" {
                  n184 = Variant To Data(error in=w251, type=FALSE, Variant=w249) -> (data=w247:bool, error out=w250:errorcluster)
                  "V10" <- w247
                  n185 = shared-variable "NI-cRIO9022-019C2C95\\Mod7\\DO0"(w247) -> ()  [unwired: 1 in, 1 out]
                }
                frame "V11" {
                  n186 = Variant To Data(error in=w256, type=FALSE, Variant=w254) -> (data=w252:bool, error out=w255:errorcluster)
                  "V11" <- w252
                  n187 = shared-variable "NI-cRIO9022-019C2C95\\Mod7\\DO1"(w252) -> ()  [unwired: 1 in, 1 out]
                }
                frame "V12" {
                  n188 = Variant To Data(error in=w261, type=FALSE, Variant=w259) -> (data=w257:bool, error out=w260:errorcluster)
                  "V12" <- w257
                  n189 = shared-variable "NI-cRIO9022-019C2C95\\Mod7\\DO2"(w257) -> ()  [unwired: 1 in, 1 out]
                }
                frame "No_Flow" {
                  w262 = FALSE
                  n190 = Variant To Data(error in=w267, type=FALSE, Variant=w265) -> (data=→"FLOW ALL OFF":bool, error out=w266:errorcluster)
                  n191 = local write "HIGH FLOW MASTER SWITCH"(w262) -> ()
                  n192 = local write "LOW FLOW MASTER SWITCH"(w262) -> ()
                }
                frame "High_Flow" {
                  w268 = FALSE
                  n193 = Variant To Data(error in=w273, type=FALSE, Variant=w271) -> (data=→"HIGH FLOW MASTER SWITCH":bool, error out=w272:errorcluster)
                  n194 = local write "LOW FLOW MASTER SWITCH"(w268) -> ()
                  n195 = local write "FLOW ALL OFF"(w268) -> ()
                }
                frame "Low_Flow" {
                  w274 = FALSE
                  n196 = Variant To Data(error in=w279, type=FALSE, Variant=w277) -> (data=→"LOW FLOW MASTER SWITCH":bool, error out=w278:errorcluster)
                  n197 = local write "HIGH FLOW MASTER SWITCH"(w274) -> ()
                  n198 = local write "FLOW ALL OFF"(w274) -> ()
                }
                frame "MFC_1" {
                  n199 = Variant To Data(error in=w284, type=0.0, Variant=w282) -> (data=w280:dbl, error out=w283:errorcluster)
                  n200 = local write "MFC_1 SLPM set value"(w280) -> ()
                }
                frame "FGGA_restart" {
                  n201 = Variant To Data(error in=w289, type=FALSE, Variant=w287) -> (data=→"FGGA restart":bool, error out=w288:errorcluster)
                }
                frame "UDP Time Offset" {
                  n202 = Variant To Data(error in=w294, type=0, Variant=w292) -> (data=→"UDP Time Stamp Offset":i32, error out=w293:errorcluster)
                }
                frame "FGGA_pump" {
                  n203 = Variant To Data(error in=w302, type=FALSE, Variant=w300) -> (data=w297:bool, error out=w301:errorcluster)
                  "FGGA Pump" <- w297
                  n204 = Select(t=1.4 ("f"), s=w297, f=0.0 ("t")) -> (s? t:f=w298:dbl)
                  n205 = shared-variable "NI-cRIO9022-019C2C95\\Mod5\\AO0"(w298) -> ()  [unwired: 1 in, 1 out]
                }
                frame "Flight Number" {
                  n206 = Variant To Data(error in=w307, type="", Variant=w305) -> (data=→"Flight Number":string, error out=w306:errorcluster)
                }
              }
            }
            frame True {
            }
          }
          n207 = node-c288() -> ()  [unwired: 1 in, 1 out]
        }
        n208 = node-c288(w191) -> ()  [unwired: 1 out]
        n209 = Destroy Stream Endpoint(8:w195, 11:w194) -> (0:→"error out 2":errorcluster)
      }
      n210 = node-c288(w45) -> ()  [unwired: 1 out]
      n211 = UDP Close(connection ID=w31, 8:w30) -> (error out=→"Labview_Viewer_UDP_Error_Out":errorcluster)  [unwired: 1 out]
      n212 = node-c288(w23) -> ()  [unwired: 1 out]
      n213 = while {
        tunnel: w42 -> [w384]
        tunnel: w41 -> [w383]
        stop <- w385 stop-if-true
        # "Must Delay to avoid 100% CPU"
        # "Broadcast FGGA UDP Data"
        n214 = call-poly <vilib>:"UDP Multicast Open.vi"("time-to-live (1)"=u16 5, "port"=u16 10000) -> ("error out"=w392:errorcluster, "connection ID"=w393:refnum<k16>)  [unwired: 8 in]
        n215 = node-c288() -> (w395:T1)  [unwired: 4 in]
        n216 = timed-loop {
          tunnel: w393 -> [w416]
          tunnel: w392 -> [w415]
          timing: w395 -> [_]
          timing-out: [_] -> w394
          shift-right: [w404] -> _
          shift-left: FALSE -> [w407]
          tunnel: [w403] -> w387
          tunnel: [w401] -> w386
          tunnel: [w399] -> w385
          tunnel: w384 -> [w397]
          tunnel: w383 -> [w396]
          stop <- w400 stop-if-true
          # "UDP Broadcast loop"
          n217 = node-c288() -> ()  [unwired: 1 in, 1 out]
          n218 = local read "Flight Number"() -> (w398:string)
          n219 = feedback-in #2(w398) -> ()
          n220 = feedback #2() -> (w409:string)  [unwired: 1 in]
          n221 = Not Equal?(x=w398, y=w409) -> (x != y?=w408:bool)
          n222 = String To IP(1:"239.1.4.6" ("name")) -> (0:w413:u32)
          n223 = flat-sequence {
            tunnel: w413 -> [w423]
            tunnel: w415 -> [w424]
            tunnel: w416 -> [w425]
            tunnel: [w425] -> w412
            tunnel: [w424] -> w411
            tunnel: [w423] -> w410
            tunnel: w408 -> [w422]
            tunnel: u16 50001 ("port or service name") -> [w436]
            tunnel: w412 -> [w435]
            tunnel: w411 -> [w434]
            tunnel: w410 -> [w433]
            tunnel: [w432] -> w403
            tunnel: [w431] -> w401
            tunnel: w397 -> [w429]
            tunnel: w396 -> [w428]
            frame #0 {
              n224 = feedback #3(u32 0) -> (w419:u32)
              n225 = case shown="False" w422 {
                tunnel: w419 -> [w426 _]
                tunnel: [w426 u32 0] -> w418
                frame False {
                }
                frame True {
                }
              }
              "UDP_Pack_num" <- w418
              n226 = Increment(x=w418) -> (x+1=w420:u32)
              n227 = feedback-in #3(w420) -> ()
            }
            frame #1 {
              n228 = Dequeue Element(queue=w429, error in (no error)=w428) -> (element=w430:string)  [unwired: 1 in, 3 out]
              n229 = UDP Write(address=w433, port or service name=w436, connection ID=w435, data in=w430, 8:w434) -> (error out=w431:errorcluster, 3:w432:refnum<k16>)  [unwired: 1 in]
            }
          }
          n230 = Select(t=FALSE, s=w407, f=TRUE) -> (s? t:f=w404:bool)
          "UDP_Out Status" <- w404
          n231 = local read "stop"() -> (w399:bool)
          n232 = node-c288() -> ()  [unwired: 1 in, 1 out]
          n233 = Unbundle(w401) -> ("status"=w402:bool)  [unwired: 2 out]
          n234 = Compound Arithmetic op=OR(w402, w399) -> (w400:bool)
        }
        n235 = node-c288(w394) -> ()  [unwired: 1 out]
        n236 = UDP Close(connection ID=w387, 8:w386) -> (error out=→"UDP_Out_Error Out":errorcluster)  [unwired: 1 out]
        n237 = Wait (ms)(milliseconds to wait=u32 1000) -> ()  [unwired: 1 out]
      }
      n238 = while {
        tunnel: w38 -> [w71]
        tunnel: w37 -> [w70]
        stop <- w74 stop-if-true
        # "Must Delay to avoid 100% CPU"
        # "TCP Loop writing to FISH Tank"
        n239 = TCP Open Connection(address="192.168.101.110", remote port or service name=u16 3502) -> (connection ID=w77:refnum<k5>, error out=w72:errorcluster)  [unwired: 3 in]
        n240 = case shown="No Error" w72 {
          selector: w72 -> [w82 w109]
          tunnel: w77 -> [w87 w110]
          tunnel: [w86 w110] -> w76
          tunnel: [w85 w109] -> w75
          tunnel: [w84 w108] -> w74
          tunnel: w71 -> [w81 _]
          tunnel: w70 -> [w80 _]
          frame No Error {
            n241 = node-c288() -> (w89:T1)  [unwired: 4 in]
            n242 = timed-loop {
              tunnel: w87 -> [w103]
              tunnel: w82 -> [w102]
              tunnel: [w101] -> w86
              tunnel: [w100] -> w85
              tunnel: [w92] -> w84
              shift-right: [w94] -> _
              shift-left: FALSE -> [w97]
              timing: w89 -> [_]
              timing-out: [_] -> w88
              tunnel: w81 -> [w91]
              tunnel: w80 -> [w90]
              stop <- w98 stop-if-true
              n243 = node-c288() -> ()  [unwired: 1 in, 1 out]
              n244 = Dequeue Element(queue=w91, error in (no error)=w90) -> (element=w93:string)  [unwired: 1 in, 3 out]
              n245 = Select(t=FALSE, s=w97, f=TRUE) -> (s? t:f=w94:bool)
              "TCP packet\nSend To FISH" <- w94
              n246 = TCP Write(connection ID=w103, data in=w93, error in (no error)=w102) -> (connection ID out=w101:refnum<k5>, error out=w100:errorcluster)  [unwired: 1 in, 1 out]
              n247 = local read "stop"() -> (w92:bool)
              n248 = Unbundle(w100) -> ("status"=w99:bool)  [unwired: 2 out]
              n249 = node-c288() -> ()  [unwired: 1 in, 1 out]
              n250 = Compound Arithmetic op=OR(w99, w92) -> (w98:bool)
            }
            n251 = node-c288(w88) -> ()  [unwired: 1 out]
          }
          frame Error {
            n252 = local read "stop"() -> (w108:bool)
          }
        }
        n253 = TCP Close Connection(connection ID=w76, error in (no error)=w75) -> (error out=→"FISH TCP Error Out":errorcluster)  [unwired: 1 in, 1 out]
        n254 = Wait (ms)(milliseconds to wait=u32 1000) -> ()  [unwired: 1 out]
      }
      n255 = while {
        tunnel: w40 -> [w113]
        tunnel: w39 -> [w112]
        stop <- w116 stop-if-true
        # "Must Delay to avoid 100% CPU"
        # "TCP Loop writing to SEPTIC Tank"
        n256 = TCP Open Connection(address="192.168.101.108", remote port or service name=u16 3502) -> (connection ID=w119:refnum<k5>, error out=w114:errorcluster)  [unwired: 3 in]
        n257 = case shown="No Error" w114 {
          selector: w114 -> [w124 w151]
          tunnel: w119 -> [w129 w152]
          tunnel: [w128 w152] -> w118
          tunnel: [w127 w151] -> w117
          tunnel: [w126 w150] -> w116
          tunnel: w113 -> [w123 _]
          tunnel: w112 -> [w122 _]
          frame No Error {
            n258 = node-c288() -> (w131:T1)  [unwired: 4 in]
            n259 = timed-loop {
              tunnel: w129 -> [w145]
              tunnel: w124 -> [w144]
              tunnel: [w143] -> w128
              tunnel: [w142] -> w127
              tunnel: [w134] -> w126
              shift-right: [w136] -> _
              shift-left: FALSE -> [w139]
              timing: w131 -> [_]
              timing-out: [_] -> w130
              tunnel: w123 -> [w133]
              tunnel: w122 -> [w132]
              stop <- w140 stop-if-true
              n260 = node-c288() -> ()  [unwired: 1 in, 1 out]
              n261 = Dequeue Element(queue=w133, error in (no error)=w132) -> (element=w135:string)  [unwired: 1 in, 3 out]
              n262 = Select(t=FALSE, s=w139, f=TRUE) -> (s? t:f=w136:bool)
              "TCP packet\nSend To SEPTIC" <- w136
              n263 = TCP Write(connection ID=w145, data in=w135, error in (no error)=w144) -> (connection ID out=w143:refnum<k5>, error out=w142:errorcluster)  [unwired: 1 in, 1 out]
              n264 = local read "stop"() -> (w134:bool)
              n265 = Unbundle(w142) -> ("status"=w141:bool)  [unwired: 2 out]
              n266 = node-c288() -> ()  [unwired: 1 in, 1 out]
              n267 = Compound Arithmetic op=OR(w141, w134) -> (w140:bool)
            }
            n268 = node-c288(w130) -> ()  [unwired: 1 out]
          }
          frame Error {
            n269 = local read "stop"() -> (w150:bool)
          }
        }
        n270 = TCP Close Connection(connection ID=w118, error in (no error)=w117) -> (error out=→"SEPTIC TCP Error Out":errorcluster)  [unwired: 1 in, 1 out]
        n271 = Wait (ms)(milliseconds to wait=u32 1000) -> ()  [unwired: 1 out]
      }
      n272 = while {
        stop <- FALSE stop-if-true
        # "Emergency shutdown on the valves when connection to the client drops"
        n273 = shared-variable ".\\Global Shared Variables.lvlib\\Disconnect_WatchDog"() -> (w49:bool)  [unwired: 1 in, 1 out]
        n274 = Wait (ms)(milliseconds to wait=u32 1000) -> ()  [unwired: 1 out]
        n275 = case shown="True" w49 {
          frame False {
          }
          frame True {
            w56 = FALSE
            n276 = local read "HIGH FLOW MASTER SWITCH"() -> (w53:bool)
            n277 = local read "LOW FLOW MASTER SWITCH"() -> (w52:bool)
            n278 = local read "FLOW ALL OFF"() -> (w54:bool)
            n279 = shared-variable "NI-cRIO9022-019C2C95\\Mod6\\DO1"(w56) -> ()  [unwired: 1 in, 1 out]
            n280 = shared-variable "NI-cRIO9022-019C2C95\\Mod6\\DO3"(w56) -> ()  [unwired: 1 in, 1 out]
            n281 = shared-variable "NI-cRIO9022-019C2C95\\Mod6\\DO0"(w56) -> ()  [unwired: 1 in, 1 out]
            n282 = shared-variable "NI-cRIO9022-019C2C95\\Mod6\\DO2"(w56) -> ()  [unwired: 1 in, 1 out]
            n283 = case shown="True" w54 {
              frame False {
              }
              frame True {
                # "Disable eV10, 11& 12 & FGGA pump"
                n284 = flat-sequence {
                  frame #0 {
                    n285 = shared-variable "NI-cRIO9022-019C2C95\\Mod5\\AO0"(0.0) -> ()  [unwired: 1 in, 1 out]
                  }
                  frame #1 {
                    n286 = shared-variable "NI-cRIO9022-019C2C95\\Mod7\\DO1"(FALSE) -> ()  [unwired: 1 in, 1 out]
                  }
                  frame #2 {
                    n287 = shared-variable "NI-cRIO9022-019C2C95\\Mod7\\DO0"(FALSE) -> ()  [unwired: 1 in, 1 out]
                  }
                  frame #3 {
                    n288 = shared-variable "NI-cRIO9022-019C2C95\\Mod7\\DO2"(FALSE) -> ()  [unwired: 1 in, 1 out]
                  }
                }
              }
            }
            n289 = case shown="True" w53 {
              frame False {
              }
              frame True {
                # "Disable FGGA pump & eV11, Enable eV10 & 12"
                n290 = flat-sequence {
                  frame #0 {
                    n291 = shared-variable "NI-cRIO9022-019C2C95\\Mod5\\AO0"(0.0) -> ()  [unwired: 1 in, 1 out]
                  }
                  frame #1 {
                    n292 = shared-variable "NI-cRIO9022-019C2C95\\Mod7\\DO1"(FALSE) -> ()  [unwired: 1 in, 1 out]
                  }
                  frame #2 {
                    n293 = shared-variable "NI-cRIO9022-019C2C95\\Mod7\\DO0"(TRUE) -> ()  [unwired: 1 in, 1 out]
                  }
                  frame #3 {
                    n294 = shared-variable "NI-cRIO9022-019C2C95\\Mod7\\DO2"(TRUE) -> ()  [unwired: 1 in, 1 out]
                  }
                }
              }
            }
            n295 = case shown="True" w52 {
              frame False {
              }
              frame True {
                # "Disable eV10 & eV12, Enable eV11 & FGGA pump"
                n296 = flat-sequence {
                  frame #0 {
                    n297 = shared-variable "NI-cRIO9022-019C2C95\\Mod7\\DO0"(FALSE) -> ()  [unwired: 1 in, 1 out]
                  }
                  frame #1 {
                    n298 = shared-variable "NI-cRIO9022-019C2C95\\Mod7\\DO2"(FALSE) -> ()  [unwired: 1 in, 1 out]
                  }
                  frame #2 {
                    n299 = shared-variable "NI-cRIO9022-019C2C95\\Mod7\\DO1"(TRUE) -> ()  [unwired: 1 in, 1 out]
                  }
                  frame #3 {
                    n300 = shared-variable "NI-cRIO9022-019C2C95\\Mod5\\AO0"(1.4) -> ()  [unwired: 1 in, 1 out]
                  }
                }
              }
            }
            n301 = local write "MFC_1 SLPM set value"(0.0 ("MFC_1 SLPM set value")) -> ()
          }
        }
      }
    }
    frame Error {
    }
  }
  n302 = VISA Close(VISA resource name=w17, error in (no error)=w18) -> (error out=→"Serial error out":errorcluster)
